vi "ProcessConfiguration.vi"(8 "error in (no error)":errorcluster) -> (0 "error out":errorcluster, 3 "config":T1)   [LabVIEW 2017, in "SinglePointClock.lvlib"]
uses:
  <vilib>/addons/InsightCM/Devices/Shared/Common/SinglePointClock/SinglePointClock.lvlib
  <vilib>/addons/InsightCM/Devices/Shared/Common/SinglePointClock/controls/SinglePointConfig.ctl
  <vilib>/addons/InsightCM/Utilities/GlobalConfiguration/GlobalConfiguration.lvlib
  <vilib>/addons/InsightCM/Utilities/DeviceModelHelpers/DeviceModelHelpers.lvlib
  <vilib>/addons/InsightCM/Utilities/PropertyHelpers/PropertyHelpers.lvlib
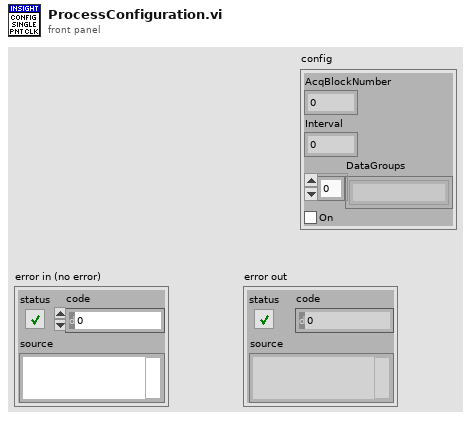
[diagram p1: front panel]
types:
  T1 = typedef "SinglePointConfig.ctl" = cluster{"AcqBlockNumber":i32, "Interval":dbl, "DataGroups":string[], "On":bool}
  T2 = typedef "SectionKeyValues.ctl" = cluster{"Section":string, "KeyValues":T3[]}
  T3 = typedef "KeyValuePair.ctl" = cluster{"Key":string, "Value":string}
  T4 = typedef "R2_DeviceModel.ctl" = cluster{"Device":T5, "Channels":T15[], "Tags":T17[]}
  T5 = typedef "R2_Device.ctl" = cluster{"Id":string, "Name":string, "DeviceType":string, "HardwareName":string, "IpAddress":string, "HardwareInfo":T3[], "ApplicationType":string, "ApplicationVersion":string, "EquipmentIds":string[], "ConfigurationVersion":string, "State":T6, "Properties":T3[], "DataGroups":T7[], "BurstModeTrigger":T11, "SensorGroups":T12[], "Endpoints":T13[]}
  T6 = typedef "DeviceState.ctl" = cluster{"Disabled":bool}
  T7 = typedef "R2_DataGroup.ctl" = cluster{"Name":string, "OperatingStates":T8[], "Properties":T3[], "EquipmentIds":string[], "AssetNodeId":string}
  T8 = typedef "OperatingState.ctl" = cluster{"Name":string, "Properties":T3[], "Triggers":T9[]}
  T9 = typedef "Trigger.ctl" = cluster{"Type":string, "Expression":string, "Conditions":T10[]}
  T10 = typedef "Condition.ctl" = cluster{"Source":string, "Type":string, "Operator":string, "CompareTo":string, "DwellSeconds":dbl}
  T11 = typedef "BurstModeTrigger.ctl" = cluster{"Trigger":T9, "SampleRate":string, "AcquisitionLength":string}
  T12 = typedef "DeviceSensorGroup.ctl" = cluster{"EquipId":string, "SensorGroupId":string}
  T13 = typedef "WirelessEndpoint.ctl" = cluster{"SerialNumber":string, "Properties":T3[], "Channels":T14[]}
  T14 = typedef "WirelessChannel.ctl" = cluster{"ChannelNumber":i32, "AssetId":string}
  T15 = typedef "R2_Channel.ctl" = cluster{"Id":string, "DeviceId":string, "Name":string, "ChannelType":string, "HardwareKey":string, "HardwareChannel":string, "DataGroup":string, "Keywords":string[], "EquipmentIds":string[], "Properties":T3[], "Metrics":T16[], "AssetNodeId":string, "MeasType":string, "AssetName":string}
  T16 = typedef "Metric.ctl" = cluster{"Id":string, "Name":string, "Unit":string, "Properties":T3[], "MetricDefinitionInstanceId":string}
  T17 = typedef "Tag.ctl" = cluster{"Id":string, "Path":string, "Name":string, "Datatype":string, "Props":T3[], "Keywords":string[]}
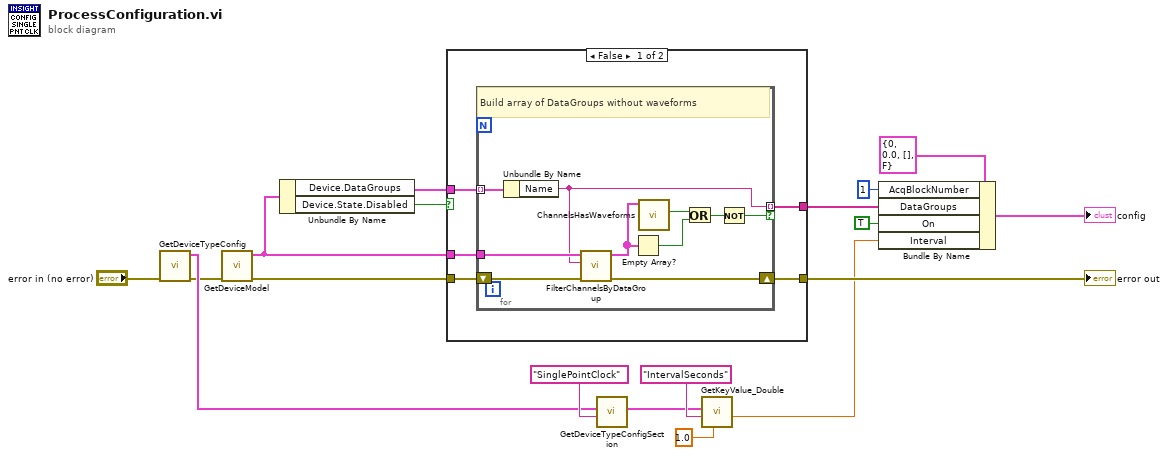
[diagram p0: block diagram]
diagram:
  n1 = call <vilib>:"GetDeviceTypeConfig.vi"("error in (no error)"="error in (no error)") -> ("error out"=w4:errorcluster, "key values"=w7:T2[])  [unwired: 8 in, 1 out]
  n2 = call <vilib>:"GetDeviceModel.vi"("error in (no error)"=w4) -> ("error out"=w6:errorcluster, "device model"=w16:T4)  [unwired: 8 in, 1 out]
  n3 = Unbundle By Name(w16) -> ("Device.DataGroups"=w18:T7[], "Device.State.Disabled"=w10:bool)
  n4 = case shown="False" w10 {
    tunnel: w18 -> [w23 _]
    tunnel: w6 -> [w22 w34]
    tunnel: [w21 w34] -> w17
    tunnel: w16 -> [w20 _]
    tunnel: [w19 _] -> w14
    frame False {
      n5 = for {
        tunnel: w23 -> [w32] mode=indexing
        shift-right: [w29] -> w21
        shift-left: w22 -> [w30]
        tunnel: [w28] -> w19 mode=indexing if=w33
        tunnel: w20 -> [w31]
        # "Build array of DataGroups without waveforms"
        n6 = Unbundle By Name(w32) -> ("Name"=w28:string)
        n7 = call <vilib>:"FilterChannelsByDataGroup.vi"("error in (no error)"=w30, "group"=w28, "device model"=w31) -> ("error out"=w29:errorcluster, "channels in data group"=w27:T15[])  [unwired: 7 in]
        n8 = Empty Array?(array=w27) -> (empty?=w26:bool)
        n9 = call <vilib>:"ChannelsHasWaveforms.vi"("channels"=w27) -> ("has waveforms"=w25:bool)  [unwired: 10 in]
        n10 = Or(x=w25, y=w26) -> (x .or. y?=w24:bool)
        n11 = Not(x=w24) -> (.not. x?=w33:bool)
      }
    }
    frame True {
    }
  }
  "error out" <- w17
  n12 = call <vilib>:"GetDeviceTypeConfigSection.vi"("key"="SinglePointClock", "key values"=w7) -> ("key value pairs out"=w3:T3[])  [unwired: 8 in, 1 out]
  n13 = call <vilib>:"GetKeyValue_Double.vi"("default"=1.0, "key"="IntervalSeconds" ("Key"), "key value pairs"=w3) -> ("value"=w1:dbl)  [unwired: 6 in, 2 out]
  n14 = Bundle By Name(cluster=T1 {"AcqBlockNumber"=0, "Interval"=0.0, "DataGroups"=[], "On"=FALSE} ("Cluster"), "AcqBlockNumber"=1, "DataGroups"=w14, "On"=TRUE, "Interval"=w1) -> (→"config":T1)
